vi "Posiciones_Alrededor_Posicion_xy.vi"(4 "Num_Columnas":dbl, 5 "Num_Filas":dbl, 7 "Posicion_Mina":string) -> (0 "Posicion_Derecha":string, 1 "Posicion_Izquierda":string, 2 "Posicion_Inferior":string, 3 "Posicion_Superior":string)   [LabVIEW 2019]
doc: "Parametros -------------------------------------\n\n'Posicion_Mina': Corresponde a una cadena de texto con una posición 'x,y' donde 'x' e 'y' son numeros enteros.\n'Num_Filas': Corresponde al número de filas limite.\n'Num_Columnas': Corresponde al número de columnas limite.\n\nRetorna ----------------------------------------\n\n'Posicion_Superior': Corresponde a una cadena de texto con la posición 'x,y' superior a la posición pasada como parametro.\n'Posicion_Inferior': Corresponde a una cadena de texto con la posición 'x,y' inferior a la posición pasada como parametro.\n'Posicion_Izquierda': Corresponde a una cadena de texto con la posición 'x,y' a la izquierda de la posición pasada como parametro.\n'Posicion_IDerecha': Corresponde a una cadena de texto con la posición 'x,y' a la derecha de la posición pasada como parametro.\n\nSe retornara una cadena en blanco si no existe la correspondiente posición."
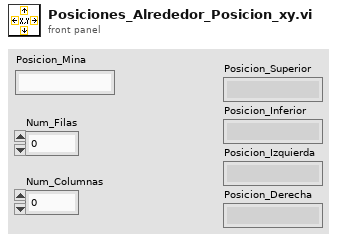
[diagram p1: front panel]
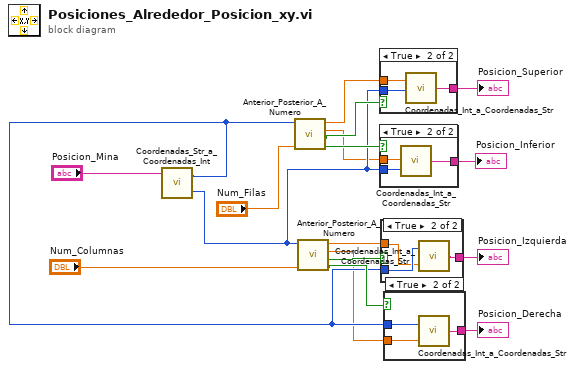
[diagram p0: block diagram]
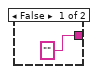
[diagram p2: hidden frame]
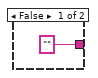
[diagram p3: hidden frame]
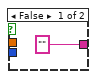
[diagram p4: hidden frame]
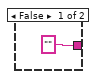
[diagram p5: hidden frame]
diagram:
  n1 = call "Coordenadas_Str_a_Coordenadas_Int.vi"("Coordenadas_Str"="Posicion_Mina") -> ("Columna"=w9:i32, "Fila"=w10:i32)  [unwired: 1 in]
  n2 = call "Anterior_Posterior_A_Numero.vi"("Limite_Superior"="Num_Filas", "Numero"=w10) -> ("Cumple_Limite_Superior"=w13:bool, "Cumple_Limite_Inferior"=w14:bool, "Posterior"=w7:dbl, "Anterior"=w8:dbl)  [unwired: 2 in]
  n3 = call "Anterior_Posterior_A_Numero.vi"("Limite_Superior"="Num_Columnas", "Numero"=w9) -> ("Cumple_Limite_Superior"=w11:bool, "Cumple_Limite_Inferior"=w12:bool, "Posterior"=w5:dbl, "Anterior"=w6:dbl)  [unwired: 2 in]
  n4 = case shown="True" w14 {
    tunnel: ["" w19] -> w4
    tunnel: w9 -> [_ w20]
    tunnel: w8 -> [_ w21]
    frame False {
    }
    frame True {
      n5 = call "Coordenadas_Int_a_Coordenadas_Str.vi"("Columna"=w20, "Fila"=w21) -> ("Posicion_str"=w19:string)
    }
  }
  "Posicion_Superior" <- w4
  n6 = case shown="True" w13 {
    tunnel: ["" w23] -> w3
    tunnel: w9 -> [_ w24]
    tunnel: w7 -> [_ w25]
    frame False {
    }
    frame True {
      n7 = call "Coordenadas_Int_a_Coordenadas_Str.vi"("Columna"=w24, "Fila"=w25) -> ("Posicion_str"=w23:string)
    }
  }
  "Posicion_Inferior" <- w3
  n8 = case shown="True" w12 {
    tunnel: ["" w29] -> w2
    tunnel: w10 -> [_ w28]
    tunnel: w6 -> [_ w27]
    frame False {
    }
    frame True {
      n9 = call "Coordenadas_Int_a_Coordenadas_Str.vi"("Columna"=w27, "Fila"=w28) -> ("Posicion_str"=w29:string)
    }
  }
  "Posicion_Izquierda" <- w2
  n10 = case shown="True" w11 {
    tunnel: ["" w33] -> w1
    tunnel: w10 -> [_ w31]
    tunnel: w5 -> [_ w32]
    frame False {
    }
    frame True {
      n11 = call "Coordenadas_Int_a_Coordenadas_Str.vi"("Columna"=w32, "Fila"=w31) -> ("Posicion_str"=w33:string)
    }
  }
  "Posicion_Derecha" <- w1
